vi "Drive Teleop Handler.vi"(10 "Call Context":T1, 11 "Manipulator Mode 2":T2) -> ()   [LabVIEW 2020]
uses:
  swerve/Type Definitions/Data/Robot Velocities.ctl
  Teleop Util/Driver Controls Mode.ctl
  <vilib>/Rock Robotics/WPI/DriverStation/WPI_DriverStationDerivedRobotMode.ctl
  Drive/Implementation/Driving Mode.ctl
  <vilib>/Rock Robotics/WPI/Joystick/XBox Buttons Indexer.ctl
  ce51abe2-3967-49ec-91df-d4b8ef358bb3.vi
  20f039dc-a6f5-4e97-88ba-31848a91c715.vi
  fdc21bd4-9215-41b8-8367-bf19dde4ba27.vi
  <vilib>/Rock Robotics/WPI/Utilities/WPI_GetSetVariantRefNum.vi
  <vilib>/Rock Robotics/Network Tables/NT Read Number.vi
  <vilib>/Rock Robotics/Network Tables/NT Read Boolean.vi
  <vilib>/Rock Robotics/Network Tables/NT Write Boolean.vi
  Framework/Robot Global Data.vi
panel:
  in  "Deadband Info":T3={"Deadband"=0.05, "Deadband High"=1.0, "Deadband Low"=0.05}
  in  "Max Velocities":T4={"X Velocity"=15.0, "Y Velocity"=15.0, "Rotational \nVelocity"=270.0}
  in  "Sinusoidal Terms":cluster{"Max Velocity":dbl, "Frequency":dbl}
  in  "Teleop Mode":T5(ring)
  in  "Joystick Inputs":T6(array[cluster])
  in  "Send Inputs":bool
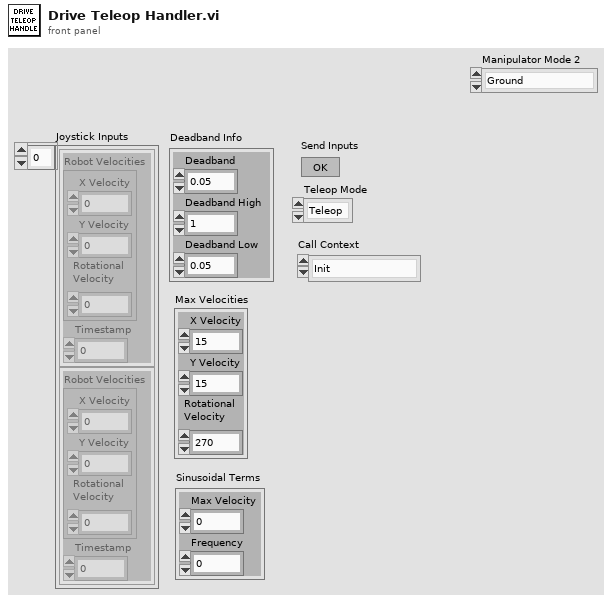
[diagram p1: front panel]
types:
  T1 = typedef "WPI_DriverStationDerivedRobotMode.ctl" = enum16{"Init", "Execute", "Stop"}
  T2 = typedef "Driver Controls Mode.ctl" = enum16{"Ground", "Scoring"}
  T3 = cluster{"Deadband":dbl, "Deadband High":dbl, "Deadband Low":dbl}
  T4 = typedef "Robot Velocities.ctl" = cluster{"X Velocity":dbl, "Y Velocity":dbl, "Rotational \nVelocity":dbl}
  T5 = enum16{"Teleop", "Simulated Teleop", "Sine Velocity Profiles", "Circle Simulator"}
  T6 = cluster{"Robot Velocities":T4, "Timestamp":dbl}[]
  T7 = typedef "Driving Mode.ctl" = enum16{"Robot Centric", "Field Centric"}
  T8 = typedef "XBox Buttons Indexer.ctl" = enum16{"A", "B", "X", "Y", "Left Bumper", "Right Bumper", "Back", "Start", "Left Joystick", "Right Joystick"}
  T9 = typedef "WPI_JoystickDevRef.ctl" = cluster{"Device":T10}
  T10 = typedef "WPI_JoystickDeviceEnum.ctl" = enum16{"USB 0", "USB 1", "USB 2", "USB 3", "USB 4", "USB 5"}
  T11 = typedef "CTRE_PigeonIMU_DeviceRef.ctl" = cluster{"DeviceStatus":errorcluster, "Device Number":u8, "Type":T12, "Device ID":u32, "Handle":u64, "UsageFrame":u32, "Library Path":path}
  T12 = typedef "CTRE_PigeonIMU_ConnectionType.ctl" = u32
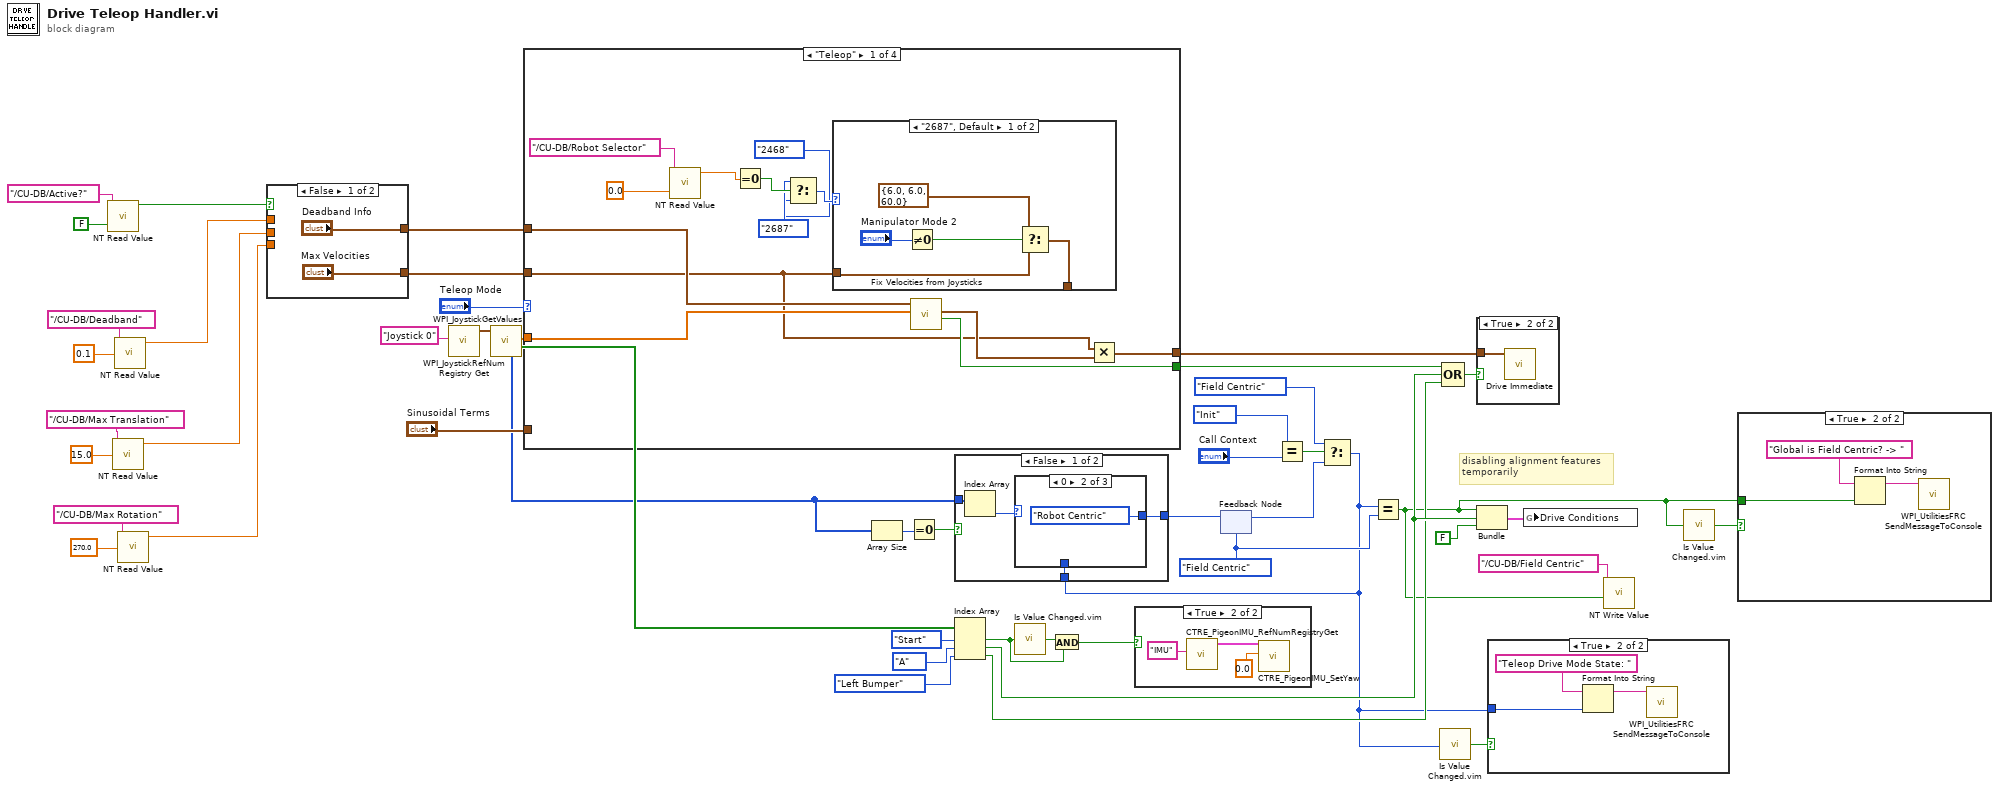
[diagram p0: block diagram]
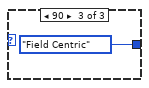
[diagram p5: hidden frame]
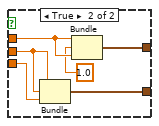
[diagram p7: hidden frame]
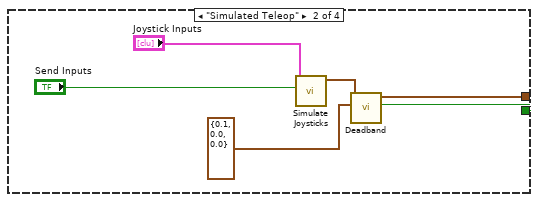
[diagram p9: hidden frame]
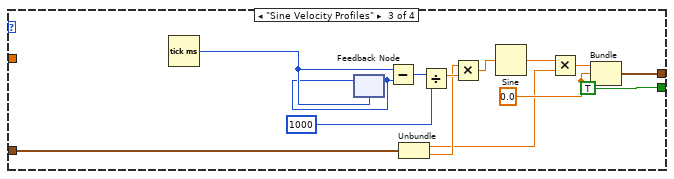
[diagram p10: hidden frame]
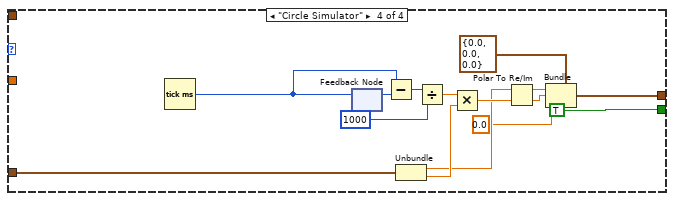
[diagram p11: hidden frame]
diagram:
  w6 = Driving_Mode."Field Centric"
  # "disabling alignment features\ntemporarily"
  n1 = call-poly <vilib>:"NT Read Value.vi"("default value"=FALSE ("Default Value"), "name"="/CU-DB/Active?" ("Name")) -> ("value"=w27:bool)  [unwired: 7 in, 2 out]
  n2 = call-poly <vilib>:"NT Read Value.vi"("default value"=15.0 ("Default Value"), "name"="/CU-DB/Max Translation" ("Name")) -> ("value"=w24:dbl)  [unwired: 7 in, 2 out]
  n3 = call-poly <vilib>:"NT Read Value.vi"("default value"=0.1 ("Default Value"), "name"="/CU-DB/Deadband" ("Name")) -> ("value"=w26:dbl)  [unwired: 7 in, 2 out]
  n4 = call-poly <vilib>:"NT Read Value.vi"("default value"=270.0 ("Default Value"), "name"="/CU-DB/Max Rotation" ("Name")) -> ("value"=w23:dbl)  [unwired: 7 in, 2 out]
  n5 = case shown="False" w27 {
    tunnel: w26 -> [_ w56]
    tunnel: ["Deadband Info" w54] -> w25
    tunnel: w24 -> [_ w53]
    tunnel: w23 -> [_ w52]
    tunnel: ["Max Velocities" w51] -> w22
    frame False {
    }
    frame True {
      n6 = Bundle("value"=w53, "value"=w53, "value"=w52) -> (w51:cluster{"value":dbl, "value":dbl, "value":dbl})  [unwired: 1 in]
      n7 = Bundle("value"=w56, "value"=1.0, "value"=w56) -> (w54:cluster{"value":dbl, "value":dbl, "value":dbl})  [unwired: 1 in]
    }
  }
  n8 = call <vilib>:"WPI_JoystickRefNum Registry Get.vi"("refnum name"="Joystick 0") -> ("JoystickDevRef"=w47:T9)  [unwired: 1 in, 9 out]
  n9 = call <vilib>:"WPI_JoystickGetValues.vi"("JoystickDevRef"=w47) -> ("Buttons"=w44:bool[], "Axes"=w46:dbl[], "POVs"=w17:i16[])  [unwired: 6 in, 2 out]
  n10 = case shown="\"Teleop\"" "Teleop Mode" {
    tunnel: w46 -> [w68 _ _ _]
    tunnel: [w69 w81 w86 w97] -> w39
    tunnel: "Sinusoidal Terms" -> [_ _ w85 w105]
    tunnel: w25 -> [w67 _ _ _]
    tunnel: w22 -> [w57 _ _ _]
    tunnel: [w65 w76 TRUE ("Sending Input?") TRUE ("Sending Input?")] -> w19
    frame "Teleop" {
      n11 = call-poly <vilib>:"NT Read Value.vi"("default value"=0.0, "name"="/CU-DB/Robot Selector") -> ("value"=w62:dbl)  [unwired: 7 in, 2 out]
      n12 = Equal To 0?(x=w62) -> (x = 0?=w61:bool)
      n13 = Select(t=enum16{"2468", "2687"}."2687", s=w61, f=enum16{"2468", "2687"}."2468") -> (s? t:f=w60:enum16{"2468", "2687"})
      n14 = case shown="\"2687\", Default" w60 {
        tunnel: w57 -> [w71 w75]
        tunnel: [w70 w75] -> _
        frame "2687", Default {
          n15 = Not Equal To 0?(x="Manipulator Mode 2") -> (x != 0?=w73:bool)
          n16 = Select(t=T4 {"X Velocity"=6.0, "Y Velocity"=6.0, "Rotational \nVelocity"=60.0}, s=w73, f=w71) -> (s? t:f=w70:T4)
        }
        frame "2468" {
        }
      }
      n17 = call "Fix Velocities from Joysticks.vi"("Axes"=w68, "Deadband"=w67) -> ("Sending Input?"=w65:bool, "Adjusted Robot Velocities"=w66:T4)  [unwired: 8 in]
      n18 = Multiply(x=w57, y=w66) -> (x*y=w69:T4)
    }
    frame "Simulated Teleop" {
      n19 = call "Simulate Joysticks.vi"("Send Inputs"="Send Inputs", "Joystick Inputs"="Joystick Inputs") -> ("Joystick Inputs"=w78:T4)  [unwired: 9 in]
      n20 = call "Deadband.vi"("Deadband Info"=T3 {"Deadband"=0.1, "Deadband High"=0.0, "Deadband Low"=0.0}, "Robot Velocities"=w78) -> ("Sending Input?"=w76:bool, "Adjusted Robot Velocities"=w81:T4)  [unwired: 8 in]
    }
    frame "Sine Velocity Profiles" {
      w94 = 0.0
      n21 = Tick Count (ms)() -> (millisecond timer value=w88:u32)
      n22 = feedback #1(w88) -> (w87:u32)
      n23 = feedback-in #1(w87) -> ()
      n24 = Subtract(x=w88, y=w87) -> (x-y=w92:u32)
      n25 = Unbundle(w85) -> ("Max Velocity"=w83:dbl, "Frequency"=w84:dbl)
      n26 = Divide(x=w92, y=u32 1000) -> (x/y=w90:dbl)
      n27 = Multiply(x=w84, y=w90) -> (x*y=w89:dbl)
      n28 = Sine(x=w89) -> (sin(x)=w93:dbl)
      n29 = Multiply(x=w93, y=w83) -> (x*y=w95:dbl)
      n30 = Bundle(w95, w94, w94) -> (w86:cluster{dbl, dbl, dbl})  [unwired: 1 in]
    }
    frame "Circle Simulator" {
      n31 = Tick Count (ms)() -> (millisecond timer value=w109:u32)
      n32 = feedback-in #2(w109) -> ()
      n33 = feedback #2() -> (w110:u32)  [unwired: 1 in]
      n34 = Subtract(x=w109, y=w110) -> (x-y=w108:u32)
      n35 = Unbundle(w105) -> ("Max Velocity"=w102:dbl, "Frequency"=w104:dbl)
      n36 = Divide(x=w108, y=u32 1000) -> (x/y=w106:dbl)
      n37 = Multiply(x=w106, y=w104) -> (x*y=w103:dbl)
      n38 = Polar To Re/Im(2:w103, 3:w102) -> (0:w100:dbl, 1:w101:dbl)
      n39 = Bundle(cluster=T4 {"X Velocity"=0.0, "Y Velocity"=0.0, "Rotational \nVelocity"=0.0} ("Robot Velocities (ft/s and deg/s)"), "X Velocity"=w101, "Y Velocity"=w100, "Rotational \nVelocity"=0.0 ("Rotational \nVelocity")) -> (w97:T4)
    }
  }
  n40 = Array Size(array=w17) -> (size(s)=w16:i32)
  n41 = Equal To 0?(x=w16) -> (x = 0?=w15:bool)
  n42 = Index Array(array=w44, index #1=XBox_Buttons_Indexer."Start" ("XBox Buttons"), index #2=XBox_Buttons_Indexer."A" ("XBox Buttons"), index #3=XBox_Buttons_Indexer."Left Bumper" ("XBox Buttons")) -> (element #1=w41:bool, element #2=w14:bool, element #3=w12:bool)
  n43 = call "Is Value Changed.vim"("value"=w41) -> ("changed or first call?"=w42:bool)
  n44 = And(x=w42, y=w41) -> (x .and. y?=w40:bool)
  n45 = case shown="True" w40 {
    frame False {
    }
    frame True {
      n46 = call <vilib>:"CTRE_PigeonIMU_RefNumRegistryGet.vi"("refnum name"="IMU") -> ("PigeonIMUDevRef"=w112:T11)  [unwired: 9 in, 1 out]
      n47 = call <vilib>:"CTRE_PigeonIMU_SetYaw.vi"("Value"=0.0, "PigeonIMUDevRef"=w112) -> ()  [unwired: 8 in, 2 out]
    }
  }
  n48 = feedback #3(w6) -> (w5:T7)
  n49 = Equal?(x=WPI_DriverStationDerivedRobotMode."Init" ("y"), y="Call Context") -> (x = y?=w8:bool)
  n50 = Select(t=Driving_Mode."Field Centric" ("x"), s=w8, f=w5) -> (s? t:f=w2:T7)
  n51 = case shown="False" w15 {
    tunnel: [w116 w121] -> w45
    tunnel: w2 -> [w115 w121]
    tunnel: w17 -> [w114 _]
    frame False {
      n52 = Index Array(array=w114) -> (element=w117:i16)  [unwired: 1 in]
      n53 = case shown="0" w117 {
        tunnel: [w118 Driving_Mode."Robot Centric" Driving_Mode."Field Centric"] -> w116
        tunnel: w115 -> [w118 _ _]
        frame -1, Default {
        }
        frame 0 {
        }
        frame 90 {
        }
      }
    }
    frame True {
    }
  }
  n54 = feedback-in #3(w45) -> ()
  n55 = Equal?(x=w2, y=w6) -> (x = y?=w3:bool)
  n56 = call "Is Value Changed.vim"("value"=w2) -> ("changed or first call?"=w1:bool)
  n57 = Compound Arithmetic op=OR(w19, w14, w12) -> (w20:bool)
  n58 = case shown="True" w20 {
    tunnel: w39 -> [_ w122]
    frame False {
    }
    frame True {
      n59 = call "Drive Immediate.vi"("Robot Velocities"=w122) -> ()  [unwired: 10 in, 1 out]
    }
  }
  n60 = Bundle(w3, w14, FALSE) -> (w13:cluster{bool, bool, bool})  [unwired: 1 in]
  n61 = case shown="True" w1 {
    tunnel: w2 -> [_ w123]
    frame False {
    }
    frame True {
      n62 = Format Into String(initial string="Teleop Drive Mode State: ", w123) -> (resulting string=w125:string)  [unwired: 2 in, 1 out]
      n63 = call <vilib>:"WPI_UtilitiesFRC SendMessageToConsole.vi"("Message"=w125) -> ()  [unwired: 14 in, 1 out]
    }
  }
  n64 = global write "Robot Global Data.vi" "Drive Conditions"(w13) -> ()
  n65 = call-poly <vilib>:"NT Write Value.vi"("value"=w3, "name"="/CU-DB/Field Centric") -> ()  [unwired: 9 in, 1 out]
  n66 = call "Is Value Changed.vim"("value"=w3) -> ("changed or first call?"=w4:bool)
  n67 = case shown="True" w4 {
    tunnel: w3 -> [_ w127]
    frame False {
    }
    frame True {
      n68 = Format Into String(initial string="Global is Field Centric? -> ", w127) -> (resulting string=w128:string)  [unwired: 2 in, 1 out]
      n69 = call <vilib>:"WPI_UtilitiesFRC SendMessageToConsole.vi"("Message"=w128) -> ()  [unwired: 14 in, 1 out]
    }
  }
